vi "IScanClose.vi"(0 "PRIORLib.IScan":refnum<k7>) -> (1 "error out":errorcluster, 2 "Return":i32)   [LabVIEW 2012]
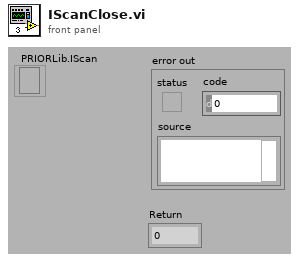
[diagram p1: front panel]
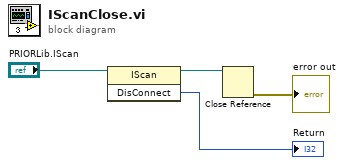
[diagram p0: block diagram]
diagram:
  n1 = invoke class="IScan" method="DisConnect"(reference="PRIORLib.IScan") -> (reference out=w4:refnum<k7>, "DisConnect"=→"Return":i32)  [unwired: 2 in, 1 out]
  n2 = Close Reference(reference=w4) -> (error out=→"error out":errorcluster)  [unwired: 1 in]
